vi "_FPGA Set PIC.vi"(4 "error in":errorcluster, 5 "Param 2":u32, 6 "Param 1":u32) -> (0 "error out":errorcluster, 3 "Data":u32)   [LabVIEW 2012]
uses:
  Type/_FPGA Indicator.ctl
  _RT Global.vi
  <vilib>/Utility/error.llb/Error Cluster From Error Code.vi
  <vilib>/rvi/errors/niLvFpgaAdjustHostInterfaceError.vi
  <vilib>/rvi/interface/nirviReadWriteControl/nirviReadWriteControl.xnode
  FPGA Bitfiles/FPGA9602.lvbitx
  NiFpgaLv.dll
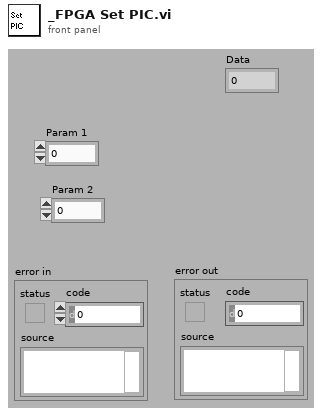
[diagram p1: front panel]
types:
  T1 = typedef "Semaphore RefNum" = refnum<k1>
  T2 = typedef "_FPGA Indicator.ctl" = enum16{"Done", "Ready", "Count Available", "SendSerial", "LED State"}
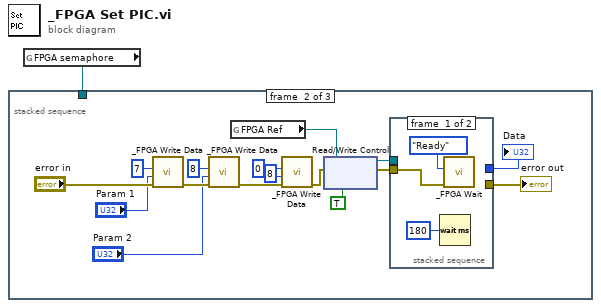
[diagram p0: block diagram]
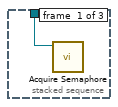
[diagram p2: hidden frame]
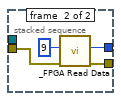
[diagram p3: hidden frame]
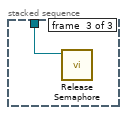
[diagram p4: hidden frame]
diagram:
  n1 = global read "_RT Global.vi" "FPGA semaphore"() -> (w1:T1)
  n2 = stacked-sequence {
    tunnel: w1 -> [w2 _ w26]
    frame #0 {
      n3 = call <vilib>:"Acquire Semaphore.vi"("semaphore"=w2) -> ()  [unwired: 2 in, 5 out]
    }
    frame #1 {
      n4 = call "_FPGA Write Data.vi"("error in"="error in", "Data"="Param 1", "Address"=u16 7) -> ("error out"=w17:errorcluster)  [unwired: 3 in, 2 out]
      n5 = call "_FPGA Write Data.vi"("error in"=w17, "Data"="Param 2", "Address"=u16 8) -> ("error out"=w8:errorcluster)  [unwired: 3 in, 2 out]
      n6 = global read "_RT Global.vi" "FPGA Ref"() -> (w3:refnum<k20>)
      n7 = call "_FPGA Write Data.vi"("error in"=w8, "Data"=u32 8 ("Address"), "Address"=u16 0) -> ("error out"=w12:errorcluster)  [unwired: 3 in, 2 out]
      n8 = xnode "Read/Write Control"("FPGA VI Reference In"=w3, "error in"=w12, "Start"=TRUE) -> ("FPGA VI Reference Out"=w6:refnum<k20>, "error out"=w7:errorcluster)
      n9 = stacked-sequence {
        tunnel: w7 -> [w19 w25]
        tunnel: w6 -> [_ _]
        tunnel: [_ w23] -> w5
        tunnel: [_ w22] -> w4
        frame #0 {
          n10 = Wait (ms)(milliseconds to wait=u32 180) -> ()  [unwired: 1 out]
          n11 = call "_FPGA Wait.vi"("error in"=w19, "Indicator"=_FPGA_Indicator."Ready") -> ()  [unwired: 3 in, 3 out]
        }
        frame #1 {
          n12 = call "_FPGA Read Data.vi"("error in"=w25, "Address"=u16 9) -> ("error out"=w23:errorcluster, "Data"=w22:u32)  [unwired: 3 in, 1 out]
        }
      }
      "error out" <- w5
      "Data" <- w4
    }
    frame #2 {
      n13 = call <vilib>:"Release Semaphore.vi"("semaphore"=w26) -> ()  [unwired: 1 in, 6 out]
    }
  }
